vi "B_SE_maker.vi"(4 "se":dbl[](array[numeric]), 6 "b":dbl[](array[numeric]), 7 "In":dbl[](array[numeric]), 9 "zeros(P,1)\nB/SE":dbl[](array[numeric]), 10 "b2":dbl[](array[numeric]), 11 "s2":dbl[](array[numeric])) -> (0 "SE":dbl[](array[numeric]), 3 "B":dbl[](array[numeric]))   [LabVIEW 2014]
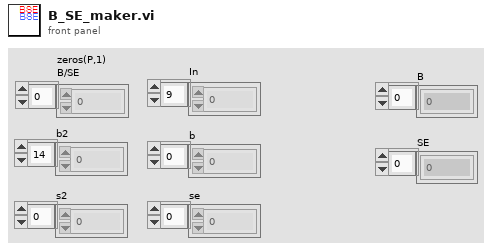
[diagram p1: front panel]
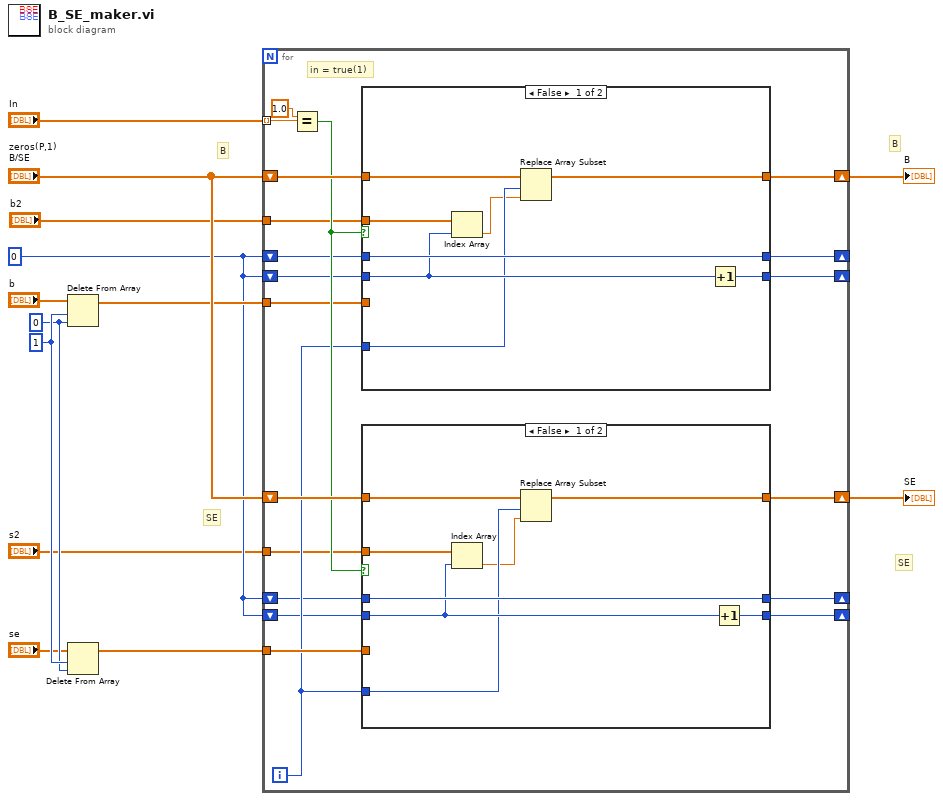
[diagram p0: block diagram]
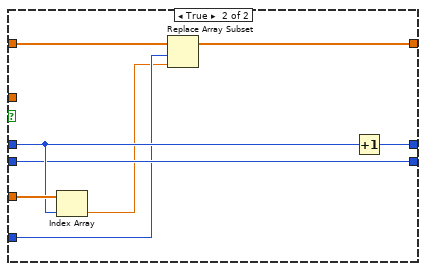
[diagram p2: hidden frame]
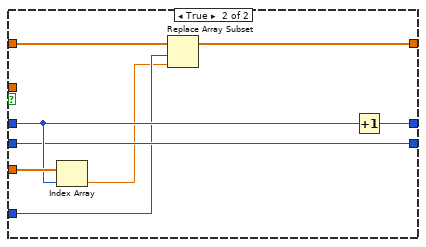
[diagram p3: hidden frame]
diagram:
  w5 = 0 ("index")
  w12 = 1 ("length")
  w11 = 0 ("index")
  # "SE"
  # "SE"
  # "B"
  # "B"
  n1 = Delete From Array(array="b", length=w12, index=w11) -> (array with subset deleted=w7:dbl[])  [unwired: 1 out]
  n2 = Delete From Array(array="se", length=w12, index=w11) -> (array with subset deleted=w6:dbl[])  [unwired: 1 out]
  n3 = for {
    shift-right: [w18] -> w2
    shift-left: "zeros(P,1)\nB/SE" -> [w33]
    shift-right: [w19] -> w1
    shift-left: "zeros(P,1)\nB/SE" -> [w32]
    tunnel: "In" -> [w31] mode=indexing
    tunnel: w7 -> [w28]
    tunnel: w6 -> [w27]
    shift-right: [w21] -> _
    shift-left: w5 -> [w25]
    shift-right: [w16] -> _
    shift-left: w5 -> [w24]
    shift-right: [w20] -> _
    shift-left: w5 -> [w23]
    shift-right: [w17] -> _
    shift-left: w5 -> [w22]
    tunnel: "b2" -> [w15]
    tunnel: "s2" -> [w14]
    i -> [w26]
    # "in = true(1)"
    n4 = Equal?(x=1.0, y=w31) -> (x = y?=w30:bool)
    n5 = case shown="False" w30 {
      tunnel: w33 -> [w55 w65]
      tunnel: w28 -> [_ w63]
      tunnel: w26 -> [w51 w59]
      tunnel: w25 -> [w57 w62]
      tunnel: w24 -> [w53 w60]
      tunnel: [w57 w64] -> w21
      tunnel: [w54 w61] -> w18
      tunnel: [w56 w60] -> w16
      tunnel: w15 -> [w52 _]
      frame False {
        n6 = Index Array(array=w52, index=w53) -> (element=w50:dbl)
        n7 = Replace Array Subset(array=w55, new element=w50, index=w51) -> (w54:dbl[])
        n8 = Increment(x=w53) -> (x+1=w56:i32)
      }
      frame True {
        n9 = Index Array(array=w63, index=w62) -> (element=w58:dbl)
        n10 = Replace Array Subset(array=w65, new element=w58, index=w59) -> (w61:dbl[])
        n11 = Increment(x=w62) -> (x+1=w64:i32)
      }
    }
    n12 = case shown="False" w30 {
      tunnel: w32 -> [w39 w49]
      tunnel: w27 -> [_ w48]
      tunnel: w26 -> [w35 w43]
      tunnel: w23 -> [w41 w46]
      tunnel: w22 -> [w37 w44]
      tunnel: [w41 w47] -> w20
      tunnel: [w38 w45] -> w19
      tunnel: [w40 w44] -> w17
      tunnel: w14 -> [w36 _]
      frame False {
        n13 = Index Array(array=w36, index=w37) -> (element=w34:dbl)
        n14 = Replace Array Subset(array=w39, new element=w34, index=w35) -> (w38:dbl[])
        n15 = Increment(x=w37) -> (x+1=w40:i32)
      }
      frame True {
        n16 = Index Array(array=w48, index=w46) -> (element=w42:dbl)
        n17 = Replace Array Subset(array=w49, new element=w42, index=w43) -> (w45:dbl[])
        n18 = Increment(x=w46) -> (x+1=w47:i32)
      }
    }
  }
  "B" <- w2
  "SE" <- w1
